vi "retrieveConfiguration.vi"(8 "error in (no error)":errorcluster, 10 "dataName":string, 11 "CompactRIO in":refnum<class "CompactRIO.lvclass">) -> (0 "error out":errorcluster, 2 "dataValueFromFile":string, 3 "CompactRIO out":refnum<class "CompactRIO.lvclass">)   [LabVIEW 2015, in "CompactRIO.lvclass"]
doc: "Retrieves the configuration data from the file associated with dataName."
uses:
  CompactRIO.lvclass
  <vilib>/Utility/xml.llb/Read From XML File.vi
  <vilib>/Utility/xml.llb/Read From XML File(string).vi
  ComponentTemplateCore/ComponentModel/ComponentModelRT/ConfigurationFileReaderRT/ConfigurationFileReaderRT.lvclass
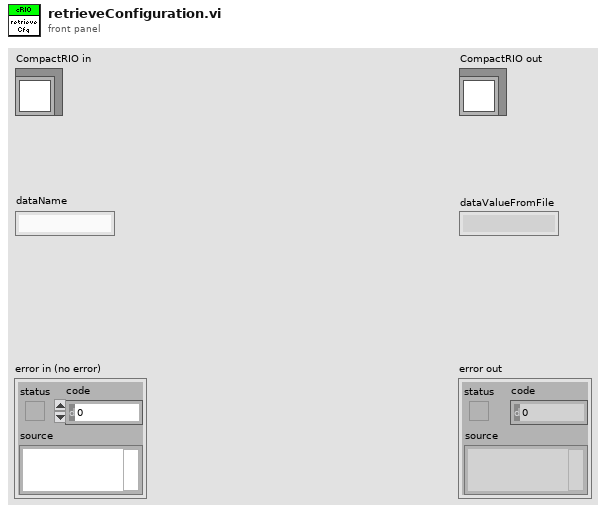
[diagram p1: front panel]
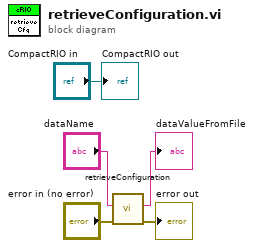
[diagram p0: block diagram]
diagram:
  n1 = call "retrieveConfiguration.vi"("error in (no error)"="error in (no error)", "dataName"="dataName") -> ("error out"=→"error out":errorcluster, "dataValueFromFile"=→"dataValueFromFile":string)  [unwired: 7 in, 1 out]
  "CompactRIO out" <- "CompactRIO in"
